vi "RTS Open Door.vi"(4 "Relay Number":u8=1 min=1 max=3 step=1, 6 "Station #":u8=1 min=1 max=8 step=1, 8 "Error In":errorcluster, 10 "Door Opening Controller Input":T1 {"Chamber 1-1"."Start Time" format="%<%X\n%x>T"; "Chamber 1-1"."End Time" format="%<%X\n%x>T"; "Time Count (s)" format="%.2f"}) -> (0 "Error Out":errorcluster, 2 "Door Opening Controller Output":T1 {"Chamber 1-1"."Start Time" format="%<%X\n%x>T"; "Chamber 1-1"."End Time" format="%<%X\n%x>T"; "Time Count (s)" format="%.2f"})   [LabVIEW 2016]
uses:
  Type Definitions/RTS Door Opener Indicator.ctl
  Type Definitions/RTS Door Ops Client.ctl
  Type Definitions/RTS Door Opening Schedule.ctl
  Type Definitions/RTS Door Ops Sequence.ctl
panel:
  out "8-3":dbl format="%.2f"
  out "8-2":dbl format="%.2f"
  out "8-1":dbl format="%.2f"
  out "7-3":dbl format="%.2f"
  out "7-2":dbl format="%.2f"
  out "7-1":dbl format="%.2f"
  out "6-3":dbl format="%.2f"
  out "6-2":dbl format="%.2f"
  out "6-1":dbl format="%.2f"
  out "5-3":dbl format="%.2f"
  out "5-2":dbl format="%.2f"
  out "5-1":dbl format="%.2f"
  out "4-3":dbl format="%.2f"
  out "4-2":dbl format="%.2f"
  out "4-1":dbl format="%.2f"
  out "3-3":dbl format="%.2f"
  out "3-2":dbl format="%.2f"
  out "3-1":dbl format="%.2f"
  out "2-3":dbl format="%.2f"
  out "2-1":dbl format="%.2f"
  out "2-2":dbl format="%.2f"
  out "1-3":dbl format="%.2f"
  out "1-2":dbl format="%.2f"
  out "1-1":dbl format="%.2f"
  # "Individual Timers"
  # "Chamber Conditions:"
  # "Chamber Conditions:"
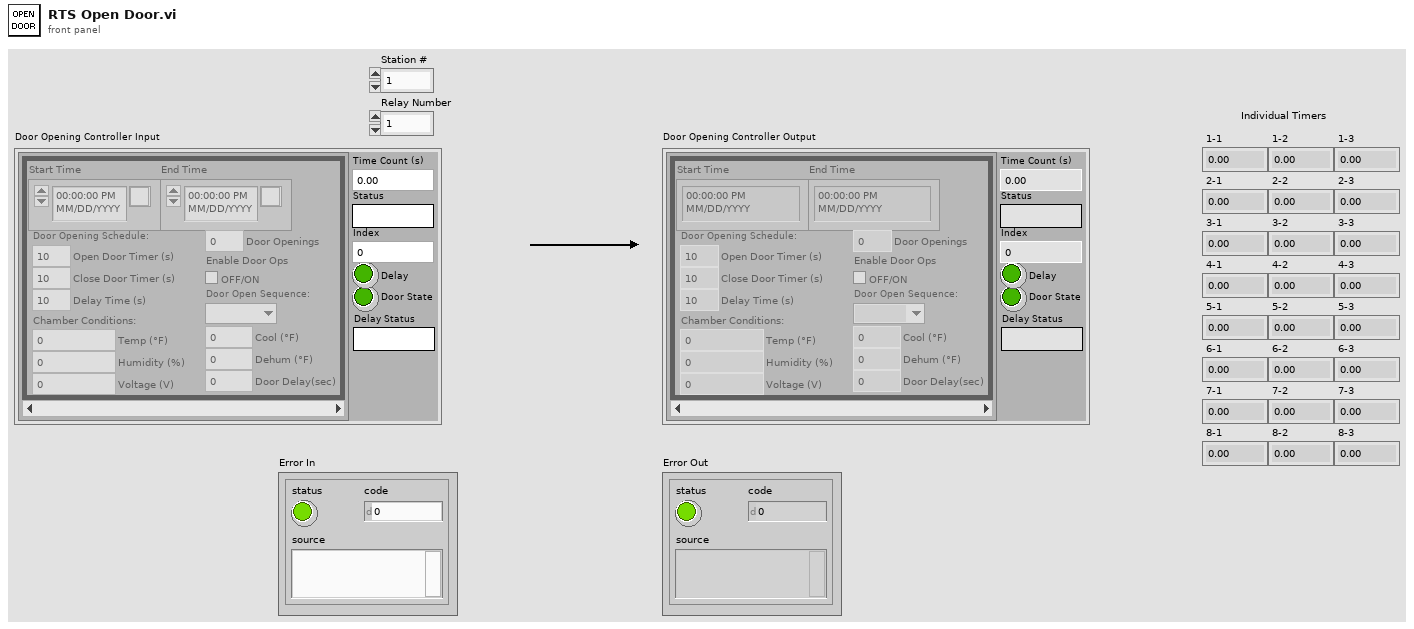
[diagram p1: front panel]
types:
  T1 = typedef "RTS Door Opener Indicator.ctl" = cluster{"Time Count (s)":dbl, "Status":string, "Door State":bool, "Delay":bool, "Chamber 1-1":T2[], "Index":i32, "Delay Status":string}
  T2 = typedef "RTS Door Ops Client.ctl" = cluster{"End Time":timestamp, "Start Time":timestamp, "Door Opening Schedule:":T3, "Enable Door Ops":bool, "Door Openings":u32, "Temp (°F)":dbl, "Humidity (%)":dbl, "Voltage (V)":dbl, "Door Open Sequence:":T4, "Door Delay(sec)":dbl, "Dehum (°F)":dbl, "Cool (°F)":dbl}
  T3 = typedef "RTS Door Opening Schedule.ctl" = cluster{"Open Door Timer (s)":dbl, "Delay Time (s)":dbl, "Close Door Timer (s)":dbl}
  T4 = typedef "RTS Door Ops Sequence.ctl" = enum16{"", "1st", "2nd", "3rd"}
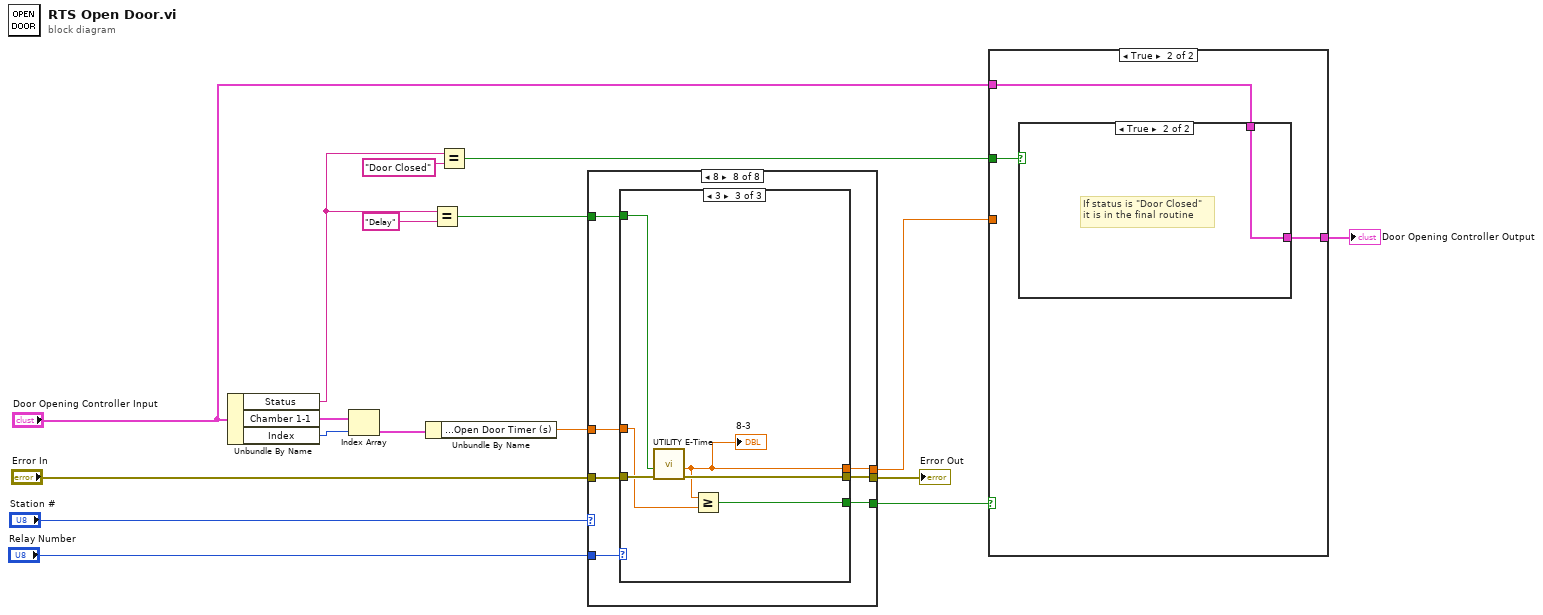
[diagram p0: block diagram]
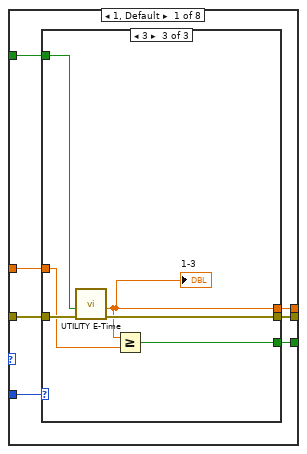
[diagram p2: hidden frame]
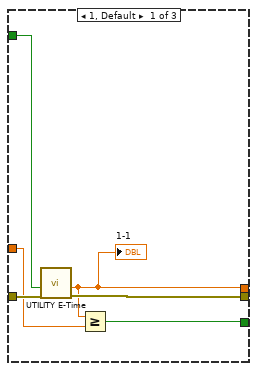
[diagram p3: hidden frame]
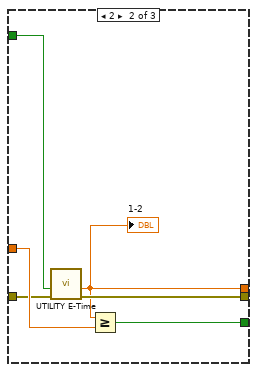
[diagram p4: hidden frame]
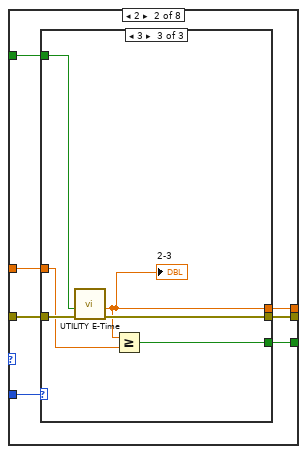
[diagram p5: hidden frame]
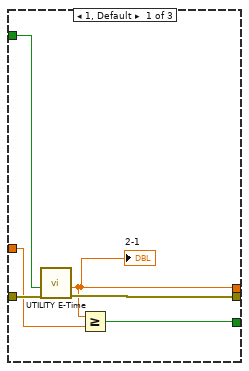
[diagram p6: hidden frame]
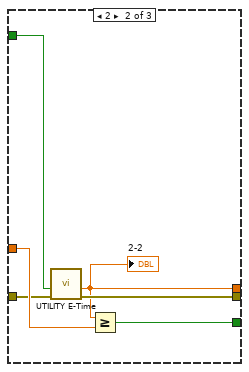
[diagram p7: hidden frame]
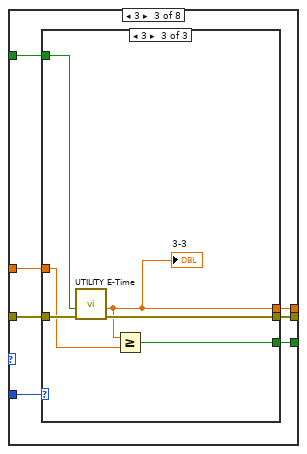
[diagram p8: hidden frame]
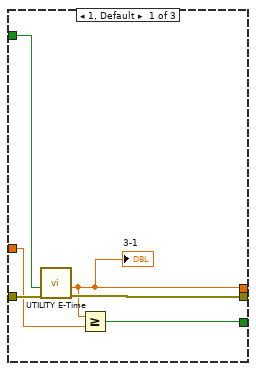
[diagram p9: hidden frame]
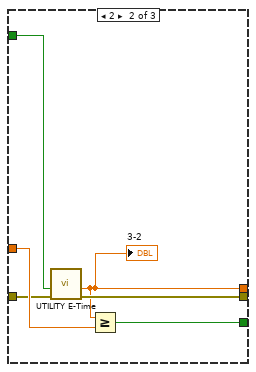
[diagram p10: hidden frame]
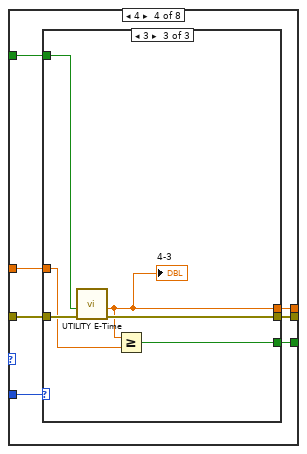
[diagram p11: hidden frame]
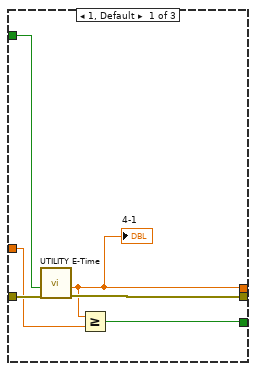
[diagram p12: hidden frame]
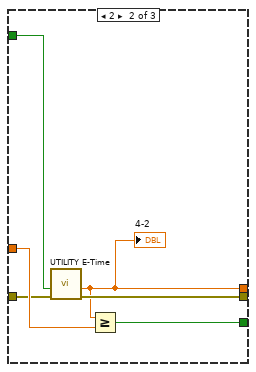
[diagram p13: hidden frame]
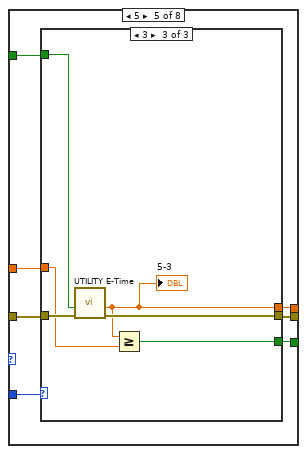
[diagram p14: hidden frame]
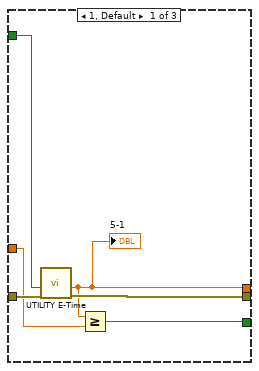
[diagram p15: hidden frame]
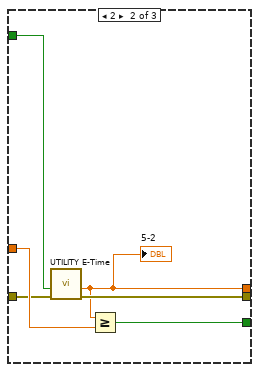
[diagram p16: hidden frame]
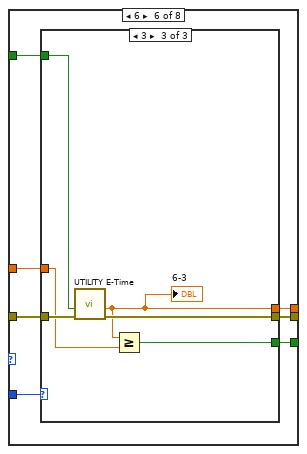
[diagram p17: hidden frame]
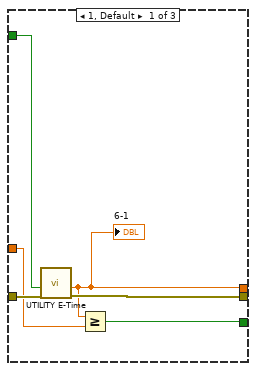
[diagram p18: hidden frame]
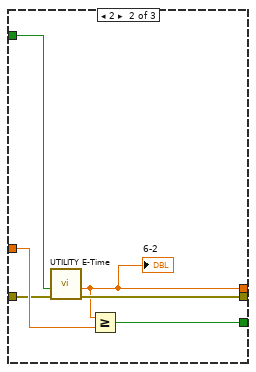
[diagram p19: hidden frame]
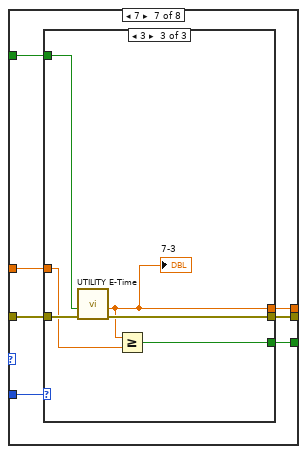
[diagram p20: hidden frame]
diagram:
  n1 = Unbundle By Name("Door Opening Controller Input") -> ("Status"=w9:string, "Chamber 1-1"=w12:T2[], "Index"=w11:i32)
  n2 = Index Array(array=w12, index=w11) -> (element=w10:T2)
  n3 = Unbundle By Name(w10) -> ("Door Opening Schedule:.Open Door Timer (s)"=w5:dbl)
  n4 = Equal?(x=w9, y="Delay") -> (x = y?=w6:bool)
  n5 = Equal?(x=w9, y="Door Closed") -> (x = y?=w14:bool)
  n6 = case shown="8" "Station #" {
    tunnel: [w24 w45 w70 w95 w120 w145 w170 w195] -> w1
    tunnel: [w23 w44 w69 w93 w118 w143 w169 w193] -> w2
    tunnel: [w22 w46 w71 w94 w119 w144 w171 w194] -> w3
    tunnel: "Error In" -> [w21 w47 w72 w97 w122 w147 w172 w197]
    tunnel: w6 -> [w20 w48 w74 w99 w124 w149 w174 w199]
    tunnel: w5 -> [w19 w43 w73 w98 w123 w148 w173 w198]
    tunnel: "Relay Number" -> [w18 w49 w68 w96 w121 w146 w168 w196]
    frame 1, Default {
      n7 = case shown="3" w18 {
        tunnel: [w28 w31 w37] -> w24
        tunnel: [w27 w34 w40] -> w23
        tunnel: [w29 w32 w41] -> w22
        tunnel: w21 -> [w30 w33 w42]
        tunnel: w20 -> [w25 w36 w38]
        tunnel: w19 -> [w26 w35 w39]
        frame 1, Default {
          n8 = call "UTILITY E-Time.vi"("error in (no error)"=w30, "Reset"=w25) -> ("error out"=w29:errorcluster, "Elapsed Time (sec)"=w28:dbl)  [unwired: 7 in, 1 out]
          "1-1" <- w28
          n9 = Greater Or Equal?(x=w28, y=w26) -> (x >= y?=w27:bool)
        }
        frame 2 {
          n10 = call "UTILITY E-Time.vi"("error in (no error)"=w33, "Reset"=w36) -> ("error out"=w32:errorcluster, "Elapsed Time (sec)"=w31:dbl)  [unwired: 7 in, 1 out]
          "1-2" <- w31
          n11 = Greater Or Equal?(x=w31, y=w35) -> (x >= y?=w34:bool)
        }
        frame 3 {
          n12 = call "UTILITY E-Time.vi"("error in (no error)"=w42, "Reset"=w38) -> ("error out"=w41:errorcluster, "Elapsed Time (sec)"=w37:dbl)  [unwired: 7 in, 1 out]
          "1-3" <- w37
          n13 = Greater Or Equal?(x=w37, y=w39) -> (x >= y?=w40:bool)
        }
      }
    }
    frame 2 {
      n14 = case shown="3" w49 {
        tunnel: [w50 w56 w62] -> w45
        tunnel: [w53 w59 w65] -> w44
        tunnel: [w54 w57 w66] -> w46
        tunnel: w47 -> [w55 w58 w67]
        tunnel: w48 -> [w51 w61 w63]
        tunnel: w43 -> [w52 w60 w64]
        frame 1, Default {
          n15 = call "UTILITY E-Time.vi"("error in (no error)"=w55, "Reset"=w51) -> ("error out"=w54:errorcluster, "Elapsed Time (sec)"=w50:dbl)  [unwired: 7 in, 1 out]
          "2-1" <- w50
          n16 = Greater Or Equal?(x=w50, y=w52) -> (x >= y?=w53:bool)
        }
        frame 2 {
          n17 = call "UTILITY E-Time.vi"("error in (no error)"=w58, "Reset"=w61) -> ("error out"=w57:errorcluster, "Elapsed Time (sec)"=w56:dbl)  [unwired: 7 in, 1 out]
          "2-2" <- w56
          n18 = Greater Or Equal?(x=w56, y=w60) -> (x >= y?=w59:bool)
        }
        frame 3 {
          n19 = call "UTILITY E-Time.vi"("error in (no error)"=w67, "Reset"=w63) -> ("error out"=w66:errorcluster, "Elapsed Time (sec)"=w62:dbl)  [unwired: 7 in, 1 out]
          "2-3" <- w62
          n20 = Greater Or Equal?(x=w62, y=w64) -> (x >= y?=w65:bool)
        }
      }
    }
    frame 3 {
      n21 = case shown="3" w68 {
        tunnel: [w75 w81 w87] -> w70
        tunnel: [w78 w84 w90] -> w69
        tunnel: [w79 w82 w91] -> w71
        tunnel: w72 -> [w80 w83 w92]
        tunnel: w74 -> [w76 w86 w88]
        tunnel: w73 -> [w77 w85 w89]
        frame 1, Default {
          n22 = call "UTILITY E-Time.vi"("error in (no error)"=w80, "Reset"=w76) -> ("error out"=w79:errorcluster, "Elapsed Time (sec)"=w75:dbl)  [unwired: 7 in, 1 out]
          "3-1" <- w75
          n23 = Greater Or Equal?(x=w75, y=w77) -> (x >= y?=w78:bool)
        }
        frame 2 {
          n24 = call "UTILITY E-Time.vi"("error in (no error)"=w83, "Reset"=w86) -> ("error out"=w82:errorcluster, "Elapsed Time (sec)"=w81:dbl)  [unwired: 7 in, 1 out]
          "3-2" <- w81
          n25 = Greater Or Equal?(x=w81, y=w85) -> (x >= y?=w84:bool)
        }
        frame 3 {
          n26 = call "UTILITY E-Time.vi"("error in (no error)"=w92, "Reset"=w88) -> ("error out"=w91:errorcluster, "Elapsed Time (sec)"=w87:dbl)  [unwired: 7 in, 1 out]
          "3-3" <- w87
          n27 = Greater Or Equal?(x=w87, y=w89) -> (x >= y?=w90:bool)
        }
      }
    }
    frame 4 {
      n28 = case shown="3" w96 {
        tunnel: [w100 w106 w112] -> w95
        tunnel: [w103 w109 w115] -> w93
        tunnel: [w104 w107 w116] -> w94
        tunnel: w97 -> [w105 w108 w117]
        tunnel: w99 -> [w101 w111 w113]
        tunnel: w98 -> [w102 w110 w114]
        frame 1, Default {
          n29 = call "UTILITY E-Time.vi"("error in (no error)"=w105, "Reset"=w101) -> ("error out"=w104:errorcluster, "Elapsed Time (sec)"=w100:dbl)  [unwired: 7 in, 1 out]
          "4-1" <- w100
          n30 = Greater Or Equal?(x=w100, y=w102) -> (x >= y?=w103:bool)
        }
        frame 2 {
          n31 = call "UTILITY E-Time.vi"("error in (no error)"=w108, "Reset"=w111) -> ("error out"=w107:errorcluster, "Elapsed Time (sec)"=w106:dbl)  [unwired: 7 in, 1 out]
          "4-2" <- w106
          n32 = Greater Or Equal?(x=w106, y=w110) -> (x >= y?=w109:bool)
        }
        frame 3 {
          n33 = call "UTILITY E-Time.vi"("error in (no error)"=w117, "Reset"=w113) -> ("error out"=w116:errorcluster, "Elapsed Time (sec)"=w112:dbl)  [unwired: 7 in, 1 out]
          "4-3" <- w112
          n34 = Greater Or Equal?(x=w112, y=w114) -> (x >= y?=w115:bool)
        }
      }
    }
    frame 5 {
      n35 = case shown="3" w121 {
        tunnel: [w125 w131 w137] -> w120
        tunnel: [w128 w134 w140] -> w118
        tunnel: [w129 w132 w141] -> w119
        tunnel: w122 -> [w130 w133 w142]
        tunnel: w124 -> [w126 w136 w138]
        tunnel: w123 -> [w127 w135 w139]
        frame 1, Default {
          n36 = call "UTILITY E-Time.vi"("error in (no error)"=w130, "Reset"=w126) -> ("error out"=w129:errorcluster, "Elapsed Time (sec)"=w125:dbl)  [unwired: 7 in, 1 out]
          "5-1" <- w125
          n37 = Greater Or Equal?(x=w125, y=w127) -> (x >= y?=w128:bool)
        }
        frame 2 {
          n38 = call "UTILITY E-Time.vi"("error in (no error)"=w133, "Reset"=w136) -> ("error out"=w132:errorcluster, "Elapsed Time (sec)"=w131:dbl)  [unwired: 7 in, 1 out]
          "5-2" <- w131
          n39 = Greater Or Equal?(x=w131, y=w135) -> (x >= y?=w134:bool)
        }
        frame 3 {
          n40 = call "UTILITY E-Time.vi"("error in (no error)"=w142, "Reset"=w138) -> ("error out"=w141:errorcluster, "Elapsed Time (sec)"=w137:dbl)  [unwired: 7 in, 1 out]
          "5-3" <- w137
          n41 = Greater Or Equal?(x=w137, y=w139) -> (x >= y?=w140:bool)
        }
      }
    }
    frame 6 {
      n42 = case shown="3" w146 {
        tunnel: [w150 w156 w162] -> w145
        tunnel: [w153 w159 w165] -> w143
        tunnel: [w154 w157 w166] -> w144
        tunnel: w147 -> [w155 w158 w167]
        tunnel: w149 -> [w151 w161 w163]
        tunnel: w148 -> [w152 w160 w164]
        frame 1, Default {
          n43 = call "UTILITY E-Time.vi"("error in (no error)"=w155, "Reset"=w151) -> ("error out"=w154:errorcluster, "Elapsed Time (sec)"=w150:dbl)  [unwired: 7 in, 1 out]
          "6-1" <- w150
          n44 = Greater Or Equal?(x=w150, y=w152) -> (x >= y?=w153:bool)
        }
        frame 2 {
          n45 = call "UTILITY E-Time.vi"("error in (no error)"=w158, "Reset"=w161) -> ("error out"=w157:errorcluster, "Elapsed Time (sec)"=w156:dbl)  [unwired: 7 in, 1 out]
          "6-2" <- w156
          n46 = Greater Or Equal?(x=w156, y=w160) -> (x >= y?=w159:bool)
        }
        frame 3 {
          n47 = call "UTILITY E-Time.vi"("error in (no error)"=w167, "Reset"=w163) -> ("error out"=w166:errorcluster, "Elapsed Time (sec)"=w162:dbl)  [unwired: 7 in, 1 out]
          "6-3" <- w162
          n48 = Greater Or Equal?(x=w162, y=w164) -> (x >= y?=w165:bool)
        }
      }
    }
    frame 7 {
      n49 = case shown="3" w168 {
        tunnel: [w175 w181 w187] -> w170
        tunnel: [w178 w184 w190] -> w169
        tunnel: [w179 w182 w191] -> w171
        tunnel: w172 -> [w180 w183 w192]
        tunnel: w174 -> [w176 w186 w188]
        tunnel: w173 -> [w177 w185 w189]
        frame 1, Default {
          n50 = call "UTILITY E-Time.vi"("error in (no error)"=w180, "Reset"=w176) -> ("error out"=w179:errorcluster, "Elapsed Time (sec)"=w175:dbl)  [unwired: 7 in, 1 out]
          "7-1" <- w175
          n51 = Greater Or Equal?(x=w175, y=w177) -> (x >= y?=w178:bool)
        }
        frame 2 {
          n52 = call "UTILITY E-Time.vi"("error in (no error)"=w183, "Reset"=w186) -> ("error out"=w182:errorcluster, "Elapsed Time (sec)"=w181:dbl)  [unwired: 7 in, 1 out]
          "7-2" <- w181
          n53 = Greater Or Equal?(x=w181, y=w185) -> (x >= y?=w184:bool)
        }
        frame 3 {
          n54 = call "UTILITY E-Time.vi"("error in (no error)"=w192, "Reset"=w188) -> ("error out"=w191:errorcluster, "Elapsed Time (sec)"=w187:dbl)  [unwired: 7 in, 1 out]
          "7-3" <- w187
          n55 = Greater Or Equal?(x=w187, y=w189) -> (x >= y?=w190:bool)
        }
      }
    }
    frame 8 {
      n56 = case shown="3" w196 {
        tunnel: [w200 w206 w212] -> w195
        tunnel: [w203 w209 w215] -> w193
        tunnel: [w204 w207 w216] -> w194
        tunnel: w197 -> [w205 w208 w217]
        tunnel: w199 -> [w201 w211 w213]
        tunnel: w198 -> [w202 w210 w214]
        frame 1, Default {
          n57 = call "UTILITY E-Time.vi"("error in (no error)"=w205, "Reset"=w201) -> ("error out"=w204:errorcluster, "Elapsed Time (sec)"=w200:dbl)  [unwired: 7 in, 1 out]
          "8-1" <- w200
          n58 = Greater Or Equal?(x=w200, y=w202) -> (x >= y?=w203:bool)
        }
        frame 2 {
          n59 = call "UTILITY E-Time.vi"("error in (no error)"=w208, "Reset"=w211) -> ("error out"=w207:errorcluster, "Elapsed Time (sec)"=w206:dbl)  [unwired: 7 in, 1 out]
          "8-2" <- w206
          n60 = Greater Or Equal?(x=w206, y=w210) -> (x >= y?=w209:bool)
        }
        frame 3 {
          n61 = call "UTILITY E-Time.vi"("error in (no error)"=w217, "Reset"=w213) -> ("error out"=w216:errorcluster, "Elapsed Time (sec)"=w212:dbl)  [unwired: 7 in, 1 out]
          "8-3" <- w212
          n62 = Greater Or Equal?(x=w212, y=w214) -> (x >= y?=w215:bool)
        }
      }
    }
  }
  "Error Out" <- w3
  n63 = case shown="True" w2 {
    tunnel: [w220 w225] -> w17
    tunnel: "Door Opening Controller Input" -> [w221 w224]
    tunnel: w1 -> [w219 _]
    tunnel: w14 -> [_ w223]
    frame False {
      n64 = Bundle By Name(cluster=w221, "Time Count (s)"=w219, "Status"="Door Open" ("Boiler Status Indicators.Status"), "Door State"=TRUE ("Gas Solenoid Valve")) -> (w220:T1)
    }
    frame True {
      n65 = case shown="True" w223 {
        tunnel: [w228 w229] -> w225
        tunnel: w224 -> [w227 w229]
        frame False {
          n66 = Bundle By Name(cluster=w227, "Status"="Door Close") -> (w228:T1)
        }
        frame True {
          # "If status is \"Door Closed\"\nit is in the final routine"
        }
      }
    }
  }
  "Door Opening Controller Output" <- w17
